vi "RT FIFO.vi"() -> ()   [LabVIEW 2015]
doc: "This application demonstrates the use of a real-time FIFO to communicate data between two loops. RT FIFOs are fixed in size, so they can communicate data between timed loops without dynamically allocating new memory. There are two FIFOs in use in this example. The first is a control FIFO that contains control information, while the other is waveform data for display. \n\nThe FIFOs in this application are used to communicate between a low priority and a high priority loop. The low priority loop reads waveform data for display on the graph and writes to the control FIFO. The high priority loop writes waveform data to the data FIFO and regulates the generated signal by reading the control FIFO.\n\nThe indicator labeled Result FIFO empty? shows whether data is remaining in the Result Data FIFO. The indicator labeled Result FIFO overwrite? shows when data in the Result Data FIFO has been lost due to an overwrite condition."
uses:
  <vilib>/Platform/TimedLoop/XDataNode/timing_clust.ctl
  <vilib>/Platform/TimedLoop/XDataNode/nitl_modes.ctl
  <vilib>/Platform/TimedLoop/XDataNode/wakeup.ctl
  <vilib>/Platform/TimedLoop/XDataNode/XDataNode.xnode
  <vilib>/Platform/TimedLoop/XDataNode/XDNodeRunTimeDep.lvlib
panel:
  out "Result FIFO overwrite?":bool
  out "Result FIFO empty?":bool
  in  "High priority rate (Hz)":dbl(slide)=250.0 scale=100.0..500.0
  in  "Low priority rate (Hz)":dbl(slide)=250.0 scale=100.0..500.0
  in  "Stop":bool
  out "Result Data":dbl(graph)=-0.7240868013690044
  in  "Amplitude":dbl(knob)=0.5048266971229651 scale=0.0..1.0 scale format="%.1f"
  # "This application demonstrates the use of a real-time FIFO to queue and communicate data between two loops.\nRT FIFOs are fixed in size, so they can communicate data between timed loops without dynamically allocating \nnew memory. There are two FIFOs in use in this example. The first is a control FIFO that contains High Priority \nLoop Rate and Amplitude control information, while the other contains waveform Result Data to display.  \n\nThe FIFOs in this application are used to communicate between a low priority and a high priority loop. The low \npriority loop reads waveform Result Data to display on the chart and writes amplitude and loop rate to the \ncontrol FIFO. The high priority loop writes waveform data to a FIFO and regulates the generated signal by \nreading the control FIFO. The indicator labeled Result FIFO empty? shows whether data is remaining in the Result \nData FIFO. The indicator labeled Result FIFO overwrite? shows when data in the Result Data FIFO is overflowing \nand has been lost due to an overwrite condition. Keep the loop rates similar to avoid these conditions."
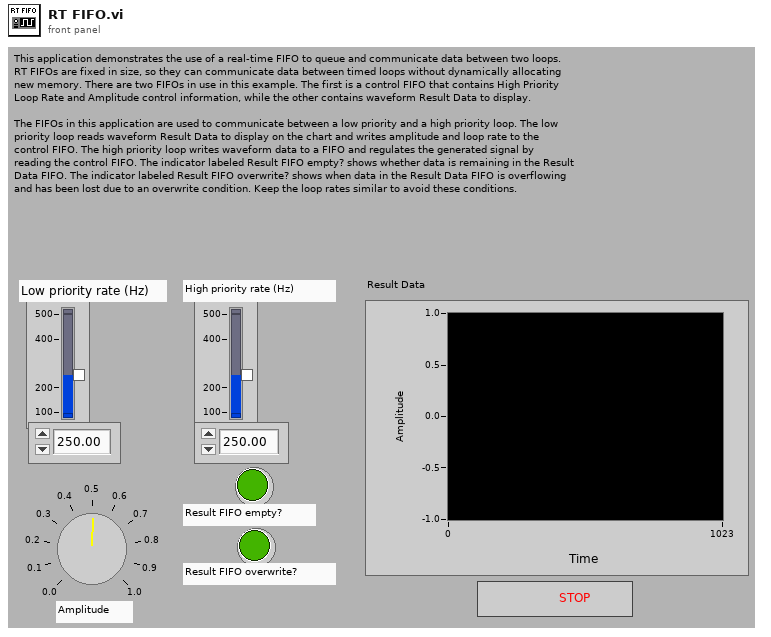
[diagram p1: front panel]
types:
  T1 = typedef "XDNodeRunTimeDep.lvlib/timing_clust.ctl" = cluster{"Expected End [f-1]":u64, "Actual End [f-1]":u64, "Finished Late? [f-1]":bool, "Expected End [i-1]":u64, "Actual End [i-1]":u64, "Finished Late? [i-1]":bool, "Expected Start [i]":u64, "Actual Start [i]":u64, "Expected Start [f]":u64, "Actual Start [f]":u64, "Source Name":string, "Structure Name":string, "Period":i64, "Deadline":i64, "Offset":i64, "Start":i64, "Priority":i32, "Timeout":i32, "Mode":T2, "Wakeup Reason":T3, "Error":errorcluster, "Source Type":string, "Secondary Source Type":string, "Global End Time":u64, "Global Start Time":u64, "Frame Duration":u64, "Iteration Duration":u64, "Assigned CPU":i32, "I/O Scan Engine Mode":u32}
  T2 = typedef "XDNodeRunTimeDep.lvlib/nitl_modes.ctl" = enum32{"No Change", "Process missed periods, maintain original phase", "Discard missed periods, maintain original phase", "Process missed periods, ignore original phase", "Discard missed periods, ignore original phase"}
  T3 = typedef "XDNodeRunTimeDep.lvlib/wakeup.ctl" = enum32{"Normal", "Aborted", "Asynchronous wakeup", "Timing source error", "Timed loop error", "Timeout"}
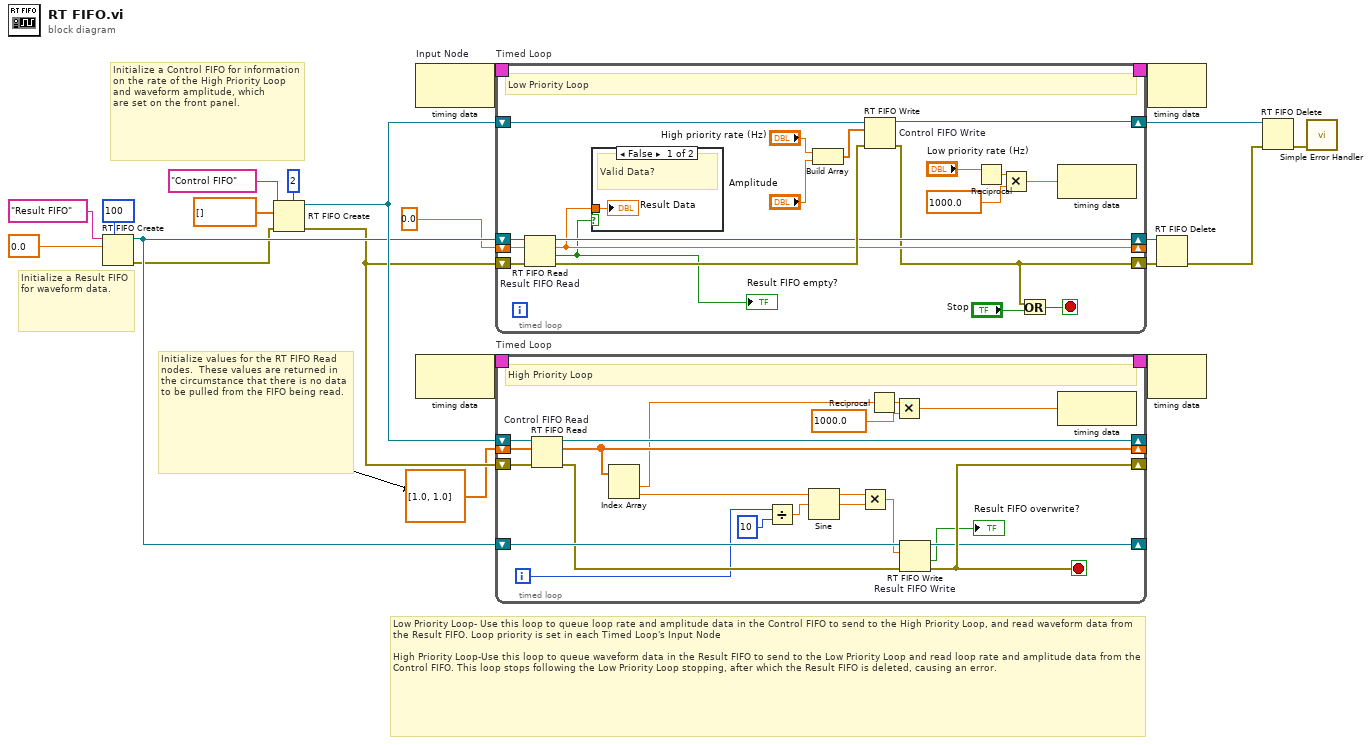
[diagram p0: block diagram]
diagram:
  # "Low Priority Loop- Use this loop to queue loop rate and amplitude data in the Control FIFO to send to the High Priority Loop, and read waveform data from the Result FIFO. Loop priority is set in each Timed Loop's Input Node\n\nHigh Priority Loop-Use this loop to queue waveform data in the Result FIFO to send to the Low Priority Loop and read loop rate and amplitude data from the Control FIFO. This loop stops following the Low Priority Loop stopping, after which the Result FIFO is deleted, causing an error."
  # "Initialize values for the RT FIFO Read nodes.  These values are returned in the circumstance that there is no data to be pulled from the FIFO being read."
  # "Initialize a Control FIFO for information on the rate of the High Priority Loop and waveform amplitude, which\nare set on the front panel."
  # "Initialize a Result FIFO for waveform data."
  n1 = RT FIFO Create(0:"Result FIFO" ("FIFO name"), 1:0.0 ("FIFO type"), 4:u32 100 ("size (10)")) -> (8:w11:refnum<k33>, 11:w10:errorcluster)  [unwired: 2 in, 4 out]
  n2 = RT FIFO Create(0:"Control FIFO" ("FIFO name"), 1:dbl[] [] ("FIFO type"), 3:w10, 6:u32 2 ("elements in array")) -> (8:w12:refnum<k33>, 11:w9:errorcluster)  [unwired: 1 in, 4 out]
  n3 = node-c288 "Input Node"() -> (w14:T1)  [unwired: 1 out]
  n4 = node-c288() -> (w5:T1)  [unwired: 1 out]
  n5 = timed-loop "Timed Loop" {
    shift-left: 0.0 ("FIFO type") -> [w38]
    shift-right: [w31] -> _
    timing: w14 -> [_]
    timing-out: [_] -> w13
    shift-right: [w22] -> w15
    shift-left: w9 -> [w39]
    shift-right: [w32] -> w18
    shift-left: w11 -> [w40]
    shift-right: [w33] -> w19
    shift-left: w12 -> [w37]
    stop <- w34 stop-if-true
    # "Low Priority Loop"
    n6 = RT FIFO Read "Result FIFO Read"(0:w40, 1:w38, 3:w39) -> (8:w32:refnum<k33>, 9:w31:dbl, 10:w26:bool, 11:w36:errorcluster)  [unwired: 2 out]
    "Result FIFO empty?" <- w26
    n7 = case shown="False" w26 {
      tunnel: w31 -> [w41 _]
      frame False {
        # "Valid Data?"
        "Result Data" <- w41
      }
      frame True {
        # "Valid Data?"
      }
    }
    n8 = Build Array("High priority rate (Hz)", "Amplitude") -> (w35:dbl[])
    n9 = RT FIFO Write "Control FIFO Write"(0:w37, 1:w35, 3:w36) -> (8:w33:refnum<k33>, 11:w22:errorcluster)  [unwired: 1 in, 3 out]
    n10 = Reciprocal(x="Low priority rate (Hz)") -> (1/x=w30:dbl)
    n11 = Multiply(x=w30, y=1000.0) -> (x*y=w27:dbl)
    n12 = Or(x=w22, y="Stop") -> (x .or. y?=w34:bool)
    n13 = node-c288(w27) -> ()  [unwired: 1 out]
  }
  n14 = timed-loop "Timed Loop" {
    shift-left: dbl[] [1.0, 1.0] -> [w64]
    shift-right: [w61] -> _
    shift-right: [w56] -> _
    shift-left: w9 -> [w53]
    shift-right: [w51] -> _
    shift-left: w11 -> [w63]
    shift-right: [w52] -> _
    shift-left: w12 -> [w65]
    timing: w5 -> [_]
    timing-out: [_] -> w4
    i -> [w49]
    stop <- w56 stop-if-true
    # "High Priority Loop"
    n15 = RT FIFO Read "Control FIFO Read"(0:w65, 1:w64, 3:w53) -> (8:w52:refnum<k33>, 9:w61:dbl[], 11:w62:errorcluster)  [unwired: 3 out]
    n16 = Index Array(array=w61) -> (element #1=w47:dbl, element #2=w46:dbl)  [unwired: 2 in]
    n17 = Divide(x=w49, y=10) -> (x/y=w59:dbl)
    n18 = Sine(x=w59) -> (sin(x)=w58:dbl)
    n19 = Multiply(x=w46, y=w58) -> (x*y=w57:dbl)
    n20 = Reciprocal(x=w47) -> (1/x=w55:dbl)
    n21 = Multiply(x=w55, y=1000.0) -> (x*y=w48:dbl)
    n22 = RT FIFO Write "Result FIFO Write"(0:w63, 1:w57, 3:w62) -> (8:w51:refnum<k33>, 10:→"Result FIFO overwrite?":bool, 11:w56:errorcluster)  [unwired: 1 in, 2 out]
    n23 = node-c288(w48) -> ()  [unwired: 1 out]
  }
  n24 = node-c288(w13) -> ()  [unwired: 1 out]
  n25 = node-c288(w4) -> ()  [unwired: 1 out]
  n26 = RT FIFO Delete(0:w18, 3:w15) -> (11:w16:errorcluster)  [unwired: 1 in]
  n27 = RT FIFO Delete(0:w19, 3:w16) -> (11:w1:errorcluster)  [unwired: 1 in]
  n28 = call <vilib>:"Simple Error Handler.vi"("error in (no error)"=w1) -> ()  [unwired: 4 in, 5 out]
